vi "Open Client Connection.vi"(8 "error in (no error)":errorcluster, 9 "Port":u16, 10 "address":string, 11 "RemoteControl.ZMQ in":refnum<class "RemoteControl.ZMQ.lvclass">) -> (0 "error out":errorcluster, 3 "RemoteControl.ZMQ out":refnum<class "RemoteControl.ZMQ.lvclass">)   [LabVIEW 2019, in "RemoteControl.ZMQ.lvclass"]
uses:
  RemoteControl.ZMQ.lvclass
  <vilib>/addons/zeromq/socket_type.ctl
  RemoteControl.ZMQ.lvclass/RemoteControl.ZMQ.ctl
  RemoteControl/RemoteControl.lvclass
  <vilib>/addons/zeromq/zmq_context.lvclass
  <vilib>/addons/zeromq/zmq_socket.lvclass
  <vilib>/addons/zeromq/zeromq.lvlib
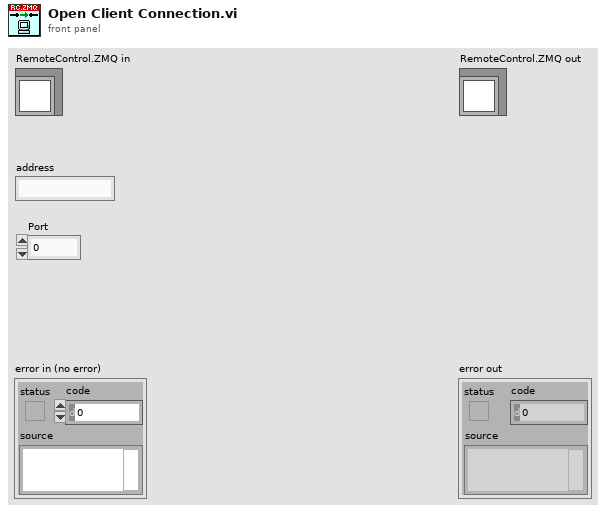
[diagram p1: front panel]
types:
  T1 = typedef "zeromq.lvlib/socket_type.ctl" = enum8{"ZMQ_PAIR", "ZMQ_PUB", "ZMQ_SUB", "ZMQ_REQ", "ZMQ_REP", "ZMQ_DEALER", "ZMQ_ROUTER", "ZMQ_PULL", "ZMQ_PUSH", "ZMQ_XPUB", "ZMQ_XSUB"}
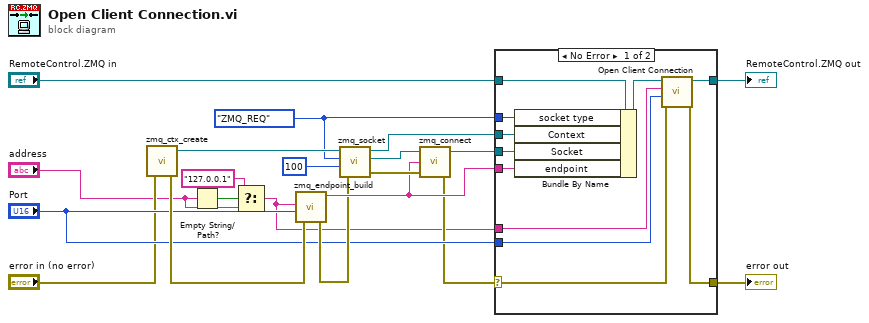
[diagram p0: block diagram]
diagram:
  w17 = socket_type."ZMQ_REQ" ("socket type")
  n1 = call <vilib>:"zmq_ctx_create.vi"("error in"="error in (no error)") -> ("error out"=w12:errorcluster, "context out"=w18:refnum<class "zmq_context.lvclass">)  [unwired: 3 in]
  n2 = Empty String/Path?(string/path="address") -> (empty?=w4:bool)
  n3 = Select(t="127.0.0.1", s=w4, f="address") -> (s? t:f=w1:string)
  n4 = call <vilib>:"zmq_endpoint_build.vi"("error in"=w12, "port"="Port", "address"=w1) -> ("error out"=w13:errorcluster, "endpoint"=w16:string)  [unwired: 2 in, 1 out]
  n5 = call <vilib>:"zmq_socket.vi"("error in"=w13, "linger (ms)"=100, "socket type"=w17, "context in"=w18) -> ("error out"=w20:errorcluster, "socket out"=w19:refnum<class "zmq_socket.lvclass">, "context out"=w15:refnum<class "zmq_context.lvclass">)  [unwired: 1 in]
  n6 = call <vilib>:"zmq_connect.vi"("error in"=w20, "endpoint"=w16, "socket in"=w19) -> ("error out"=w5:errorcluster, "socket out"=w11:refnum<class "zmq_socket.lvclass">)  [unwired: 1 in]
  n7 = case shown="No Error" w5 {
    selector: w5 -> [w21 w33]
    tunnel: w17 -> [w31 _]
    tunnel: w16 -> [w30 _]
    tunnel: w15 -> [w29 _]
    tunnel: w11 -> [w28 _]
    tunnel: w1 -> [w26 _]
    tunnel: "Port" -> [w25 _]
    tunnel: [w24 w33] -> w8
    tunnel: "RemoteControl.ZMQ in" -> [w23 w32]
    tunnel: [w22 w32] -> w6
    frame No Error {
      n8 = Bundle By Name(cluster=w23, "socket type"=w31, "Context"=w29, "Socket"=w28, "endpoint"=w30) -> (w27:refnum<class "RemoteControl.ZMQ.lvclass">)
      n9 = call-parent "Open Client Connection.vi"("error in (no error)"=w21, "Port"=w25, "address"=w26, "RemoteControl in"=w27) -> ("error out"=w24:errorcluster, "RemoteControl out"=w22:refnum<class "RemoteControl.ZMQ.lvclass">)  [unwired: 6 in]
    }
    frame Error {
    }
  }
  "error out" <- w8
  "RemoteControl.ZMQ out" <- w6
